vi "GET CHECK OUT INFO.vi"(11 "Enum":T1) -> (2 "LOCATION OUT":string, 3 "DUE DATE OUT":string)   [LabVIEW 2019]
uses:
  Controls/General Check Out Options.ctl
  <vilib>/addons/database/Connection.llb/DB Tools Open Connec (String).vi
  <vilib>/addons/database/_DB Variant To Data/Database Variant To Data.xnode
  <vilib>/addons/database/NI_Database_API.lvlib
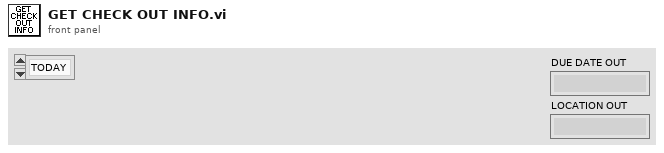
[diagram p1: front panel]
types:
  T1 = typedef "General Check Out Options.ctl" = enum16{"TODAY", "END OF SEMESTER", "MEASUREMENTS", "MECHATRONICS", "STATICS"}
  T2 = typedef "NI_Database_API.lvlib/Conn ObjectReference.ctl" = refnum<k1>
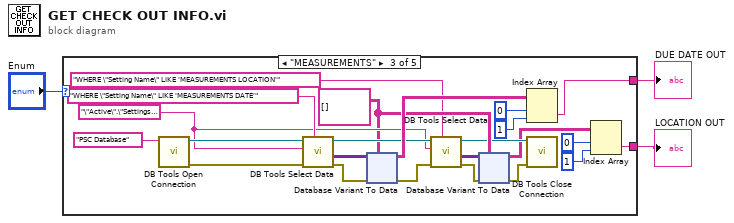
[diagram p0: block diagram]
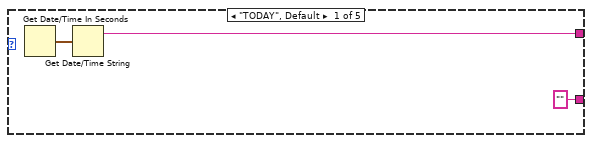
[diagram p2: hidden frame]
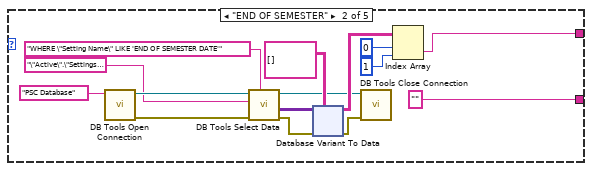
[diagram p3: hidden frame]
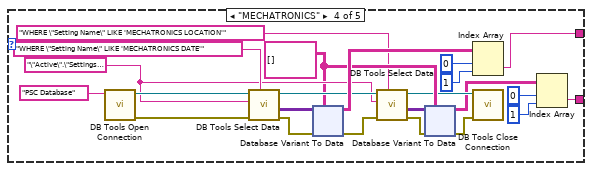
[diagram p4: hidden frame]
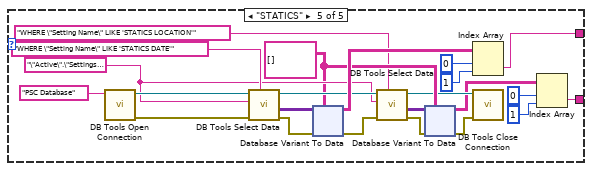
[diagram p5: hidden frame]
diagram:
  n1 = case shown="\"MEASUREMENTS\"" "Enum" {
    tunnel: [w5 w10 w79 w190 w301] -> w2
    tunnel: ["" "" w66 w177 w288] -> w1
    frame "TODAY", Default {
      n2 = Get Date/Time In Seconds() -> (seconds since 1Jan1904=w6:timestamp)
      n3 = Get Date/Time String(seconds (now)=w6) -> (date string=w5:string)  [unwired: 2 in, 1 out]
    }
    frame "END OF SEMESTER" {
      n4 = call-poly <vilib>:"DB Tools Open Connection.vi"("connection information"="PSC Database") -> ("error out"=w20:errorcluster, "connection reference"=w19:T2)  [unwired: 7 in]
      n5 = call <vilib>:"DB Tools Select Data.vi"("condition"="WHERE \"Setting Name\" LIKE 'END OF SEMESTER DATE'", "error in (no error)"=w20, "table"="\"Active\".\"Settings\"", "connection reference"=w19) -> ("error out"=w16:errorcluster, "data"=w15:variant[][], "connection reference out"=w9:T2)  [unwired: 2 in]
      n6 = xnode "Database Variant To Data"("database variant"=w15, "error in (no error)"=w16, "type"=string[][] []) -> ("data"=w13:string[][], "error out"=w8:errorcluster)
      n7 = call <vilib>:"DB Tools Close Connection.vi"("error in (no error)"=w8, "connection reference"=w9) -> ()  [unwired: 5 in, 1 out]
      n8 = Index Array(array=w13, index (row)=0, index (col)=1 ("disabled index (col)")) -> (element=w10:string)
    }
    frame "MEASUREMENTS" {
      w73 = string[][] []
      w76 = "\"Active\".\"Settings\""
      n9 = call-poly <vilib>:"DB Tools Open Connection.vi"("connection information"="PSC Database") -> ("error out"=w88:errorcluster, "connection reference"=w87:T2)  [unwired: 7 in]
      n10 = call <vilib>:"DB Tools Select Data.vi"("condition"="WHERE \"Setting Name\" LIKE 'MEASUREMENTS DATE'", "error in (no error)"=w88, "table"=w76, "connection reference"=w87) -> ("error out"=w86:errorcluster, "data"=w85:variant[][], "connection reference out"=w78:T2)  [unwired: 2 in]
      n11 = xnode "Database Variant To Data"("database variant"=w85, "error in (no error)"=w86, "type"=w73) -> ("data"=w84:string[][], "error out"=w77:errorcluster)
      n12 = call <vilib>:"DB Tools Select Data.vi"("condition"="WHERE \"Setting Name\" LIKE 'MEASUREMENTS LOCATION'", "error in (no error)"=w77, "table"=w76, "connection reference"=w78) -> ("error out"=w74:errorcluster, "data"=w75:variant[][], "connection reference out"=w71:T2)  [unwired: 2 in]
      n13 = xnode "Database Variant To Data"("database variant"=w75, "error in (no error)"=w74, "type"=w73) -> ("data"=w69:string[][], "error out"=w72:errorcluster)
      n14 = Index Array(array=w84, index (row)=0, index (col)=1 ("disabled index (col)")) -> (element=w79:string)
      n15 = call <vilib>:"DB Tools Close Connection.vi"("error in (no error)"=w72, "connection reference"=w71) -> ()  [unwired: 5 in, 1 out]
      n16 = Index Array(array=w69, index (row)=0, index (col)=1 ("disabled index (col)")) -> (element=w66:string)
    }
    frame "MECHATRONICS" {
      w184 = string[][] []
      w187 = "\"Active\".\"Settings\""
      n17 = call-poly <vilib>:"DB Tools Open Connection.vi"("connection information"="PSC Database") -> ("error out"=w199:errorcluster, "connection reference"=w198:T2)  [unwired: 7 in]
      n18 = call <vilib>:"DB Tools Select Data.vi"("condition"="WHERE \"Setting Name\" LIKE 'MECHATRONICS DATE'", "error in (no error)"=w199, "table"=w187, "connection reference"=w198) -> ("error out"=w197:errorcluster, "data"=w196:variant[][], "connection reference out"=w189:T2)  [unwired: 2 in]
      n19 = xnode "Database Variant To Data"("database variant"=w196, "error in (no error)"=w197, "type"=w184) -> ("data"=w195:string[][], "error out"=w188:errorcluster)
      n20 = call <vilib>:"DB Tools Select Data.vi"("condition"="WHERE \"Setting Name\" LIKE 'MECHATRONICS LOCATION'", "error in (no error)"=w188, "table"=w187, "connection reference"=w189) -> ("error out"=w185:errorcluster, "data"=w186:variant[][], "connection reference out"=w182:T2)  [unwired: 2 in]
      n21 = xnode "Database Variant To Data"("database variant"=w186, "error in (no error)"=w185, "type"=w184) -> ("data"=w180:string[][], "error out"=w183:errorcluster)
      n22 = Index Array(array=w195, index (row)=0, index (col)=1 ("disabled index (col)")) -> (element=w190:string)
      n23 = call <vilib>:"DB Tools Close Connection.vi"("error in (no error)"=w183, "connection reference"=w182) -> ()  [unwired: 5 in, 1 out]
      n24 = Index Array(array=w180, index (row)=0, index (col)=1 ("disabled index (col)")) -> (element=w177:string)
    }
    frame "STATICS" {
      w295 = string[][] []
      w298 = "\"Active\".\"Settings\""
      n25 = call-poly <vilib>:"DB Tools Open Connection.vi"("connection information"="PSC Database") -> ("error out"=w310:errorcluster, "connection reference"=w309:T2)  [unwired: 7 in]
      n26 = call <vilib>:"DB Tools Select Data.vi"("condition"="WHERE \"Setting Name\" LIKE 'STATICS DATE'", "error in (no error)"=w310, "table"=w298, "connection reference"=w309) -> ("error out"=w308:errorcluster, "data"=w307:variant[][], "connection reference out"=w300:T2)  [unwired: 2 in]
      n27 = xnode "Database Variant To Data"("database variant"=w307, "error in (no error)"=w308, "type"=w295) -> ("data"=w306:string[][], "error out"=w299:errorcluster)
      n28 = call <vilib>:"DB Tools Select Data.vi"("condition"="WHERE \"Setting Name\" LIKE 'STATICS LOCATION'", "error in (no error)"=w299, "table"=w298, "connection reference"=w300) -> ("error out"=w296:errorcluster, "data"=w297:variant[][], "connection reference out"=w293:T2)  [unwired: 2 in]
      n29 = xnode "Database Variant To Data"("database variant"=w297, "error in (no error)"=w296, "type"=w295) -> ("data"=w291:string[][], "error out"=w294:errorcluster)
      n30 = Index Array(array=w306, index (row)=0, index (col)=1 ("disabled index (col)")) -> (element=w301:string)
      n31 = call <vilib>:"DB Tools Close Connection.vi"("error in (no error)"=w294, "connection reference"=w293) -> ()  [unwired: 5 in, 1 out]
      n32 = Index Array(array=w291, index (row)=0, index (col)=1 ("disabled index (col)")) -> (element=w288:string)
    }
  }
  "DUE DATE OUT" <- w2
  "LOCATION OUT" <- w1
